vi "readVar.vi"(8 "错误输入（无错误）":errorcluster, 9 "var":string, 10 "id":u16, 11 "TCP网络连接输入":refnum<k5>) -> (0 "错误输出":errorcluster, 1 "data out":string, 3 "TCP网络连接输出":refnum<k5>)   [LabVIEW 2015, in "labOpenShowVar.lvlib"]
uses:
  labOpenShowVar.lvlib
panel:
  out "无符号字节数组":u8[](array[numeric])
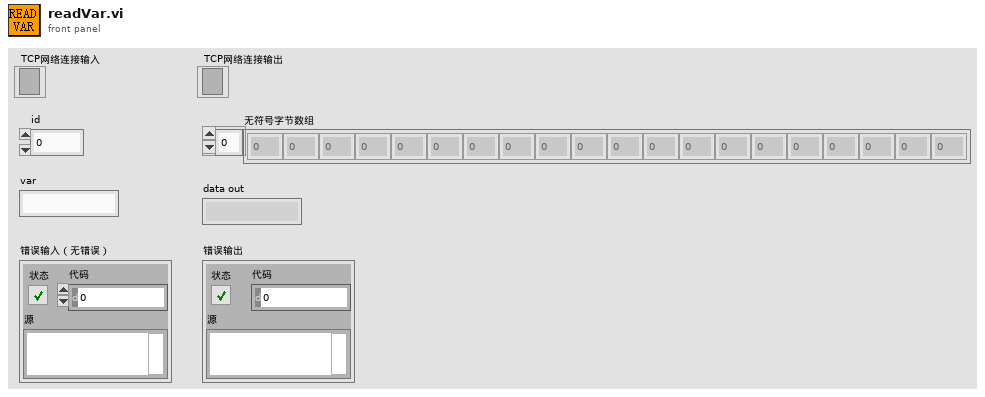
[diagram p1: front panel]
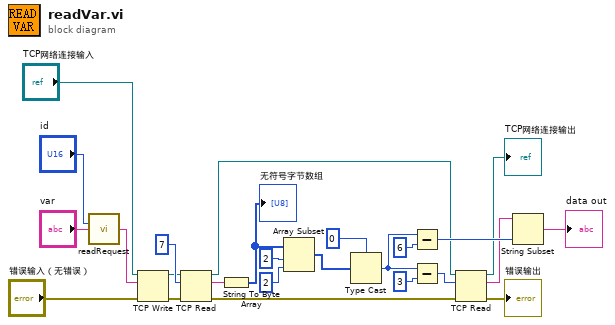
[diagram p0: block diagram]
diagram:
  n1 = call "readRequest.vi"("id"="id", "cmd"="var") -> ("readRequest"=w4:string)  [unwired: 13 in]
  n2 = TCP Write(connection ID="TCP网络连接输入", data in=w4, error in (no error)="错误输入（无错误）") -> (connection ID out=w6:refnum<k5>, error out=w7:errorcluster)  [unwired: 1 in, 1 out]
  n3 = TCP Read(connection ID=w6, bytes to read=7 ("读取的字节"), error in (no error)=w7) -> (connection ID out=w14:refnum<k5>, data out=w9:string, error out=w15:errorcluster)  [unwired: 2 in]
  n4 = String To Byte Array(string=w9) -> (unsigned byte array=w18:u8[])
  "无符号字节数组" <- w18
  n5 = Array Subset(array=w18, index=2 ("索引"), length=2 ("长度")) -> (w12:u8[])
  n6 = Type Cast(type=i16 0, x=w12) -> (*(type *) &x=w23:i16)
  n7 = Subtract(x=w23, y=i16 6) -> (x-y=w21:i16)
  n8 = Subtract(x=w23, y=i16 3) -> (x-y=w19:i16)
  n9 = TCP Read(connection ID=w14, bytes to read=w19, error in (no error)=w15) -> (connection ID out=→"TCP网络连接输出":refnum<k5>, data out=w20:string, error out=→"错误输出":errorcluster)  [unwired: 2 in]
  n10 = String Subset(string=w20, length (rest)=w21) -> (substring=→"data out":string)  [unwired: 1 in]
